vi "5492_Change_Mode.vi"(10 "Control Mode":T6=enum."Unchanged / Invalid", 11 "RobotDriveDevRef":T1={"DevStatus"={"status"=FALSE, "code"=0, "source"=""}, "Motors[]"=[], "Square Inputs"=FALSE, "Max Output"=1.0}) -> (3 "RobotDriveDevRef":T1={"DevStatus"={"status"=FALSE, "code"=0, "source"=""}, "Motors[]"=[], "Square Inputs"=FALSE, "Max Output"=1.0})   [LabVIEW 2016]
uses:
  <vilib>/Rock Robotics/WPI/RobotDrive/WPI_RobotDriveDevRef.ctl
  <vilib>/Rock Robotics/WPI/MotorControl/WPI_MotorControlDeviceRef.ctl
  <vilib>/Rock Robotics/WPI/MotorControl/WPI_MotorControlType.ctl
  <vilib>/Rock Robotics/SystemInterfaces/DIO/FPGA_DIOPWMChannel.ctl
  <vilib>/Rock Robotics/WPI/PWM/WPI_PWMDeadband.ctl
  <vilib>/Rock Robotics/WPI/ThirdParty/CanMotor/TalonSRX/WPI_CANTalonSRX_APIControlMode.ctl
  5492_WPI_RobotDriveMotorSelectorEnum.ctl
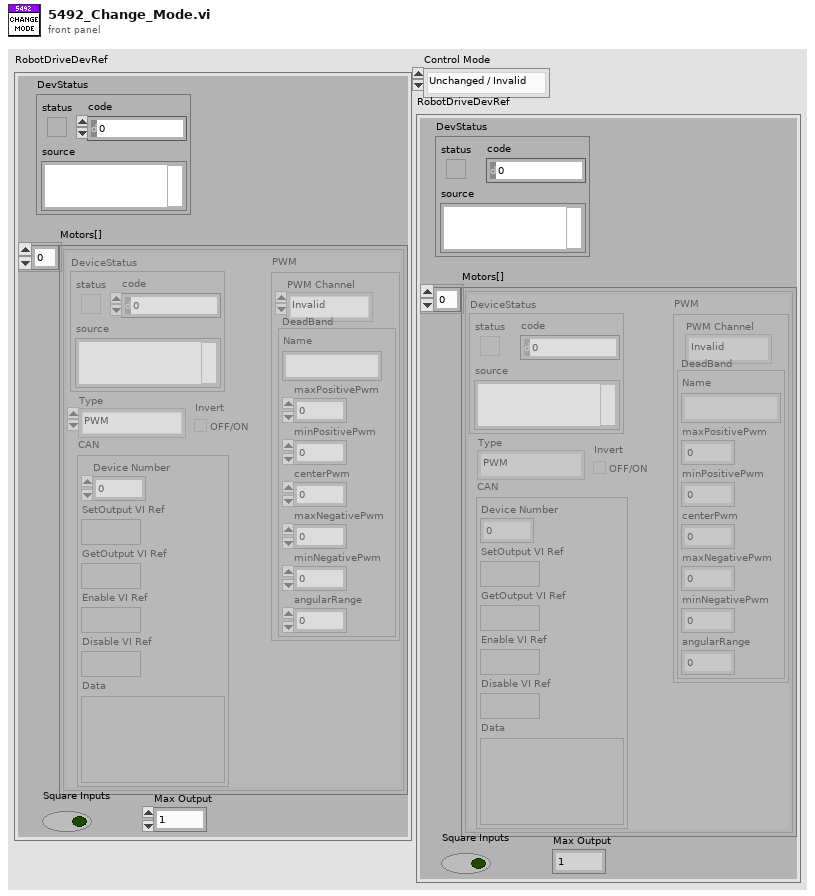
[diagram p1: front panel]
types:
  T1 = typedef "WPI_RobotDriveDevRef.ctl" = cluster{"DevStatus":errorcluster, "Motors[]":T2[], "Square Inputs":bool, "Max Output":dbl}
  T2 = typedef "WPI_MotorControlDeviceRef.ctl" = cluster{"DeviceStatus":errorcluster, "Type":T3, "PWM":cluster{"PWM Channel":T4, "DeadBand":T5}, "CAN":cluster{"Device Number":u8, "SetOutput VI Ref":variant, "GetOutput VI Ref":variant, "Enable VI Ref":variant, "Disable VI Ref":variant, "Data":variant}, "Invert":bool}
  T3 = typedef "WPI_MotorControlType.ctl" = enum16{"PWM", "CAN"}
  T4 = typedef "FPGA_DIOPWMChannel.ctl" = enum8{"PWM 0", "PWM 1", "PWM 2", "PWM 3", "PWM 4", "PWM 5", "PWM 6", "PWM 7", "PWM 8", "PWM 9", "PWM MXP 0", "PWM MXP 1", "PWM MXP 2", "PWM MXP 3", "PWM MXP 4", "PWM MXP 5", "PWM MXP 6", "PWM MXP 7", "PWM MXP 8", "PWM MXP 9", "Invalid"}
  T5 = typedef "WPI_PWMDeadband.ctl" = cluster{"Name":string, "maxPositivePwm":i32, "minPositivePwm":i32, "centerPwm":i32, "maxNegativePwm":i32, "minNegativePwm":i32, "angularRange":u16}
  T6 = typedef "WPI_CANTalonSRX_APIControlMode.ctl" = enum8{"Percent VBus", "Speed", "Position", "Slave", "Unchanged / Invalid", "Voltage Compensation", "Current", "Motion Profile", "Motion Magic"}
  T7 = typedef "5492_WPI_RobotDriveMotorSelectorEnum.ctl" = enum16{"Front left motor", "Front right motor", "Back left motor", "Back right motor", "Middle left motor", "Middle right motor"}
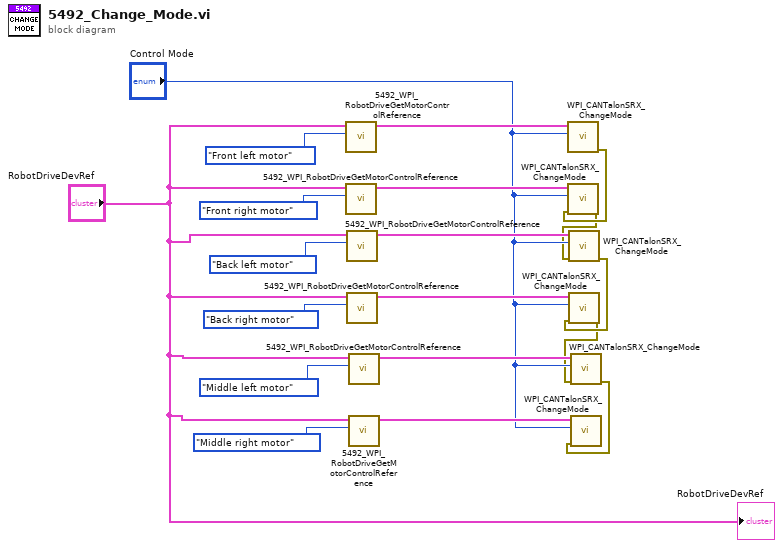
[diagram p0: block diagram]
diagram:
  n1 = call "5492_WPI_RobotDriveGetMotorControlReference.vi"("MotorIndex"=5492_WPI_RobotDriveMotorSelectorEnum."Front left motor", "RobotDriveDevRef"="RobotDriveDevRef") -> ("MotorControlDeviceRef"=w17:T2)  [unwired: 9 out]
  n2 = call "5492_WPI_RobotDriveGetMotorControlReference.vi"("MotorIndex"=5492_WPI_RobotDriveMotorSelectorEnum."Front right motor", "RobotDriveDevRef"="RobotDriveDevRef") -> ("MotorControlDeviceRef"=w16:T2)  [unwired: 9 out]
  n3 = call "5492_WPI_RobotDriveGetMotorControlReference.vi"("MotorIndex"=5492_WPI_RobotDriveMotorSelectorEnum."Back left motor", "RobotDriveDevRef"="RobotDriveDevRef") -> ("MotorControlDeviceRef"=w12:T2)  [unwired: 9 out]
  n4 = call "5492_WPI_RobotDriveGetMotorControlReference.vi"("MotorIndex"=5492_WPI_RobotDriveMotorSelectorEnum."Back right motor", "RobotDriveDevRef"="RobotDriveDevRef") -> ("MotorControlDeviceRef"=w13:T2)  [unwired: 9 out]
  n5 = call "5492_WPI_RobotDriveGetMotorControlReference.vi"("MotorIndex"=5492_WPI_RobotDriveMotorSelectorEnum."Middle left motor", "RobotDriveDevRef"="RobotDriveDevRef") -> ("MotorControlDeviceRef"=w7:T2)  [unwired: 9 out]
  n6 = call "5492_WPI_RobotDriveGetMotorControlReference.vi"("MotorIndex"=5492_WPI_RobotDriveMotorSelectorEnum."Middle right motor", "RobotDriveDevRef"="RobotDriveDevRef") -> ("MotorControlDeviceRef"=w6:T2)  [unwired: 9 out]
  n7 = call <vilib>:"WPI_CANTalonSRX_ChangeMode.vi"("Control Mode"="Control Mode", "CAN Talon SRX Ref"=w17) -> ("error out"=w15:errorcluster)  [unwired: 8 in, 1 out]
  n8 = call <vilib>:"WPI_CANTalonSRX_ChangeMode.vi"("error in (no error)"=w15, "Control Mode"="Control Mode", "CAN Talon SRX Ref"=w16) -> ("error out"=w2:errorcluster)  [unwired: 7 in, 1 out]
  n9 = call <vilib>:"WPI_CANTalonSRX_ChangeMode.vi"("error in (no error)"=w2, "Control Mode"="Control Mode", "CAN Talon SRX Ref"=w12) -> ("error out"=w14:errorcluster)  [unwired: 7 in, 1 out]
  n10 = call <vilib>:"WPI_CANTalonSRX_ChangeMode.vi"("error in (no error)"=w14, "Control Mode"="Control Mode", "CAN Talon SRX Ref"=w13) -> ("error out"=w1:errorcluster)  [unwired: 7 in, 1 out]
  n11 = call <vilib>:"WPI_CANTalonSRX_ChangeMode.vi"("error in (no error)"=w1, "Control Mode"="Control Mode", "CAN Talon SRX Ref"=w7) -> ("error out"=w5:errorcluster)  [unwired: 7 in, 1 out]
  n12 = call <vilib>:"WPI_CANTalonSRX_ChangeMode.vi"("error in (no error)"=w5, "Control Mode"="Control Mode", "CAN Talon SRX Ref"=w6) -> ()  [unwired: 7 in, 2 out]
  "RobotDriveDevRef" <- "RobotDriveDevRef"
